vi "Convert Binary to Block Data.vi"(8 "error in (no error)":errorcluster, 10 "Measurement Binary Data (\"\")":string, 11 "VISA resource name":refnum<visa-resource-name>) -> (0 "error out":errorcluster, 1 "Number of Blocks":i32, 2 "Measurement Block Data":string[](array[string]), 3 "VISA resource name out":refnum<visa-resource-name>, 4 "Number of Bytes":i32)   [LabVIEW 2020, in "Yokogawa GX Series.lvlib"]
doc: "This VI converts Measurement Binary Data to array of Blocks."
uses:
  <instrlib>/Yokogawa GX Series/Yokogawa GX Series.lvlib
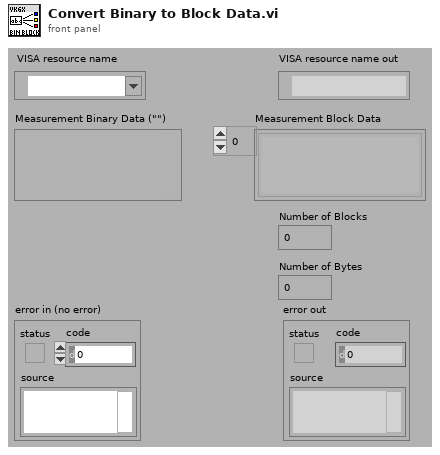
[diagram p1: front panel]
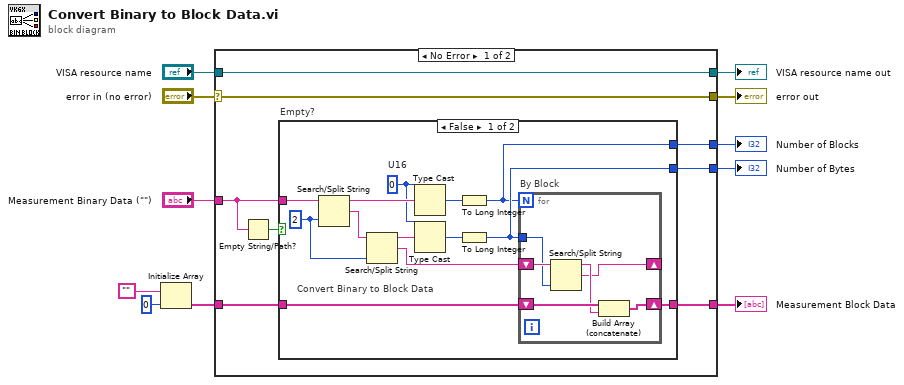
[diagram p0: block diagram]
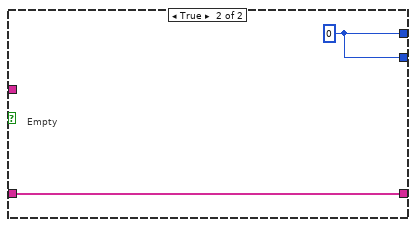
[diagram p2: hidden frame]
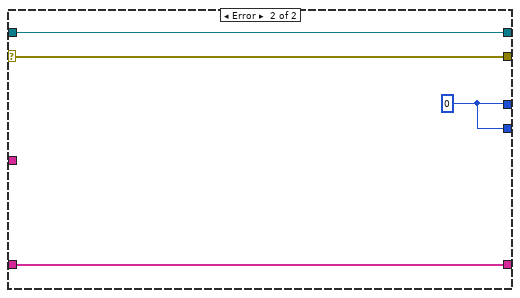
[diagram p3: hidden frame]
diagram:
  n1 = Initialize Array("", 0) -> (w9:string[])
  n2 = case shown="No Error" "error in (no error)" {
    selector: "error in (no error)" -> [w15 w43]
    tunnel: w9 -> [w19 w41]
    tunnel: "Measurement Binary Data (\"\")" -> [w12 _]
    tunnel: [w18 w41] -> w7
    tunnel: [w17 w42] -> w6
    tunnel: [w16 w42] -> w5
    tunnel: [w15 w43] -> w3
    tunnel: "VISA resource name" -> [w14 w44]
    tunnel: [w14 w44] -> w1
    frame No Error {
      n3 = Empty String/Path?(string/path=w12) -> (empty?=w13:bool)
      n4 = case "Empty?" shown="False" w13 {
        tunnel: w19 -> [w32 w40]
        tunnel: [w31 w40] -> w18
        tunnel: w12 -> [w30 _]
        tunnel: [w20 w39] -> w17
        tunnel: [w21 w39] -> w16
        frame False {
          w26 = u8 2
          w24 = u16 0  # U16
          # "Convert Binary to Block Data"
          n5 = Search/Split String(string=w30, offset (0)=w26) -> (substring before match=w28:string, match + rest of string=w29:string)  [unwired: 2 out]
          n6 = Search/Split String(string=w29, offset (0)=w26) -> (substring before match=w27:string, match + rest of string=w25:string)  [unwired: 2 out]
          n7 = Type Cast(type=w24, x=w28) -> (*(type *) &x=w23:u16)
          n8 = Type Cast(type=w24, x=w27) -> (*(type *) &x=w22:u16)
          n9 = To Long Integer(number=w23) -> (32bit integer=w20:i32)
          n10 = To Long Integer(number=w22) -> (32bit integer=w21:i32)
          n11 = for "By Block" {
            N: w20 -> [_]
            shift-right: [w37] -> w31
            shift-left: w32 -> [w38]
            tunnel: w21 -> [w33]
            shift-right: [w34] -> _
            shift-left: w25 -> [w36]
            n12 = Search/Split String(string=w36, offset (0)=w33) -> (substring before match=w35:string, match + rest of string=w34:string)  [unwired: 2 out]
            n13 = Build Array (concatenate)(w38, w35) -> (w37:string[])
          }
        }
        frame True {
          w39 = 0 ("U16")
          # "Empty"
        }
      }
    }
    frame Error {
      w42 = 0
    }
  }
  "error out" <- w3
  "VISA resource name out" <- w1
  "Measurement Block Data" <- w7
  "Number of Blocks" <- w6
  "Number of Bytes" <- w5
